vi "ceciLV_tanques.vi"() -> ()   [LabVIEW 2017]
panel:
  out "Tanque B":i64(slide) scale=0.0..100.0
  out "Tanque A":i64(slide) scale=0.0..100.0
  out "Tanque abastecimiento":i64(slide) scale=0.0..200.0
  in  "Presione despues de su seleccion:":bool
  in  "Seleccione el tanque a llenar:":u16(ring) items=["Tanque A", "Tanque B", ""]
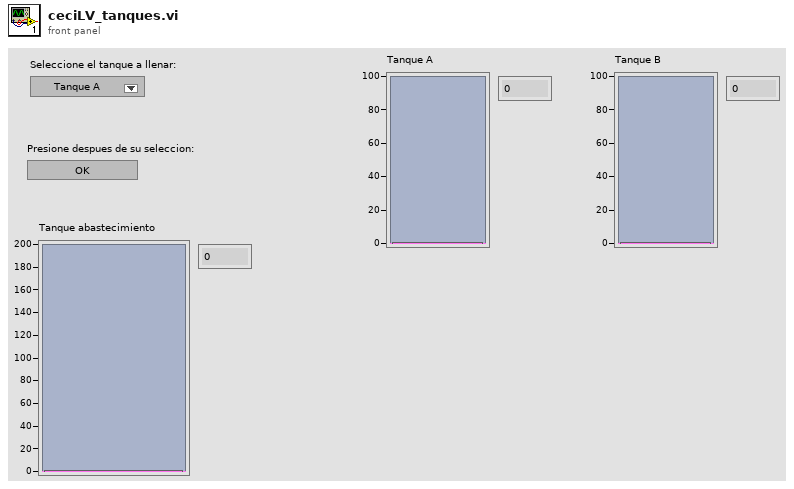
[diagram p1: front panel]
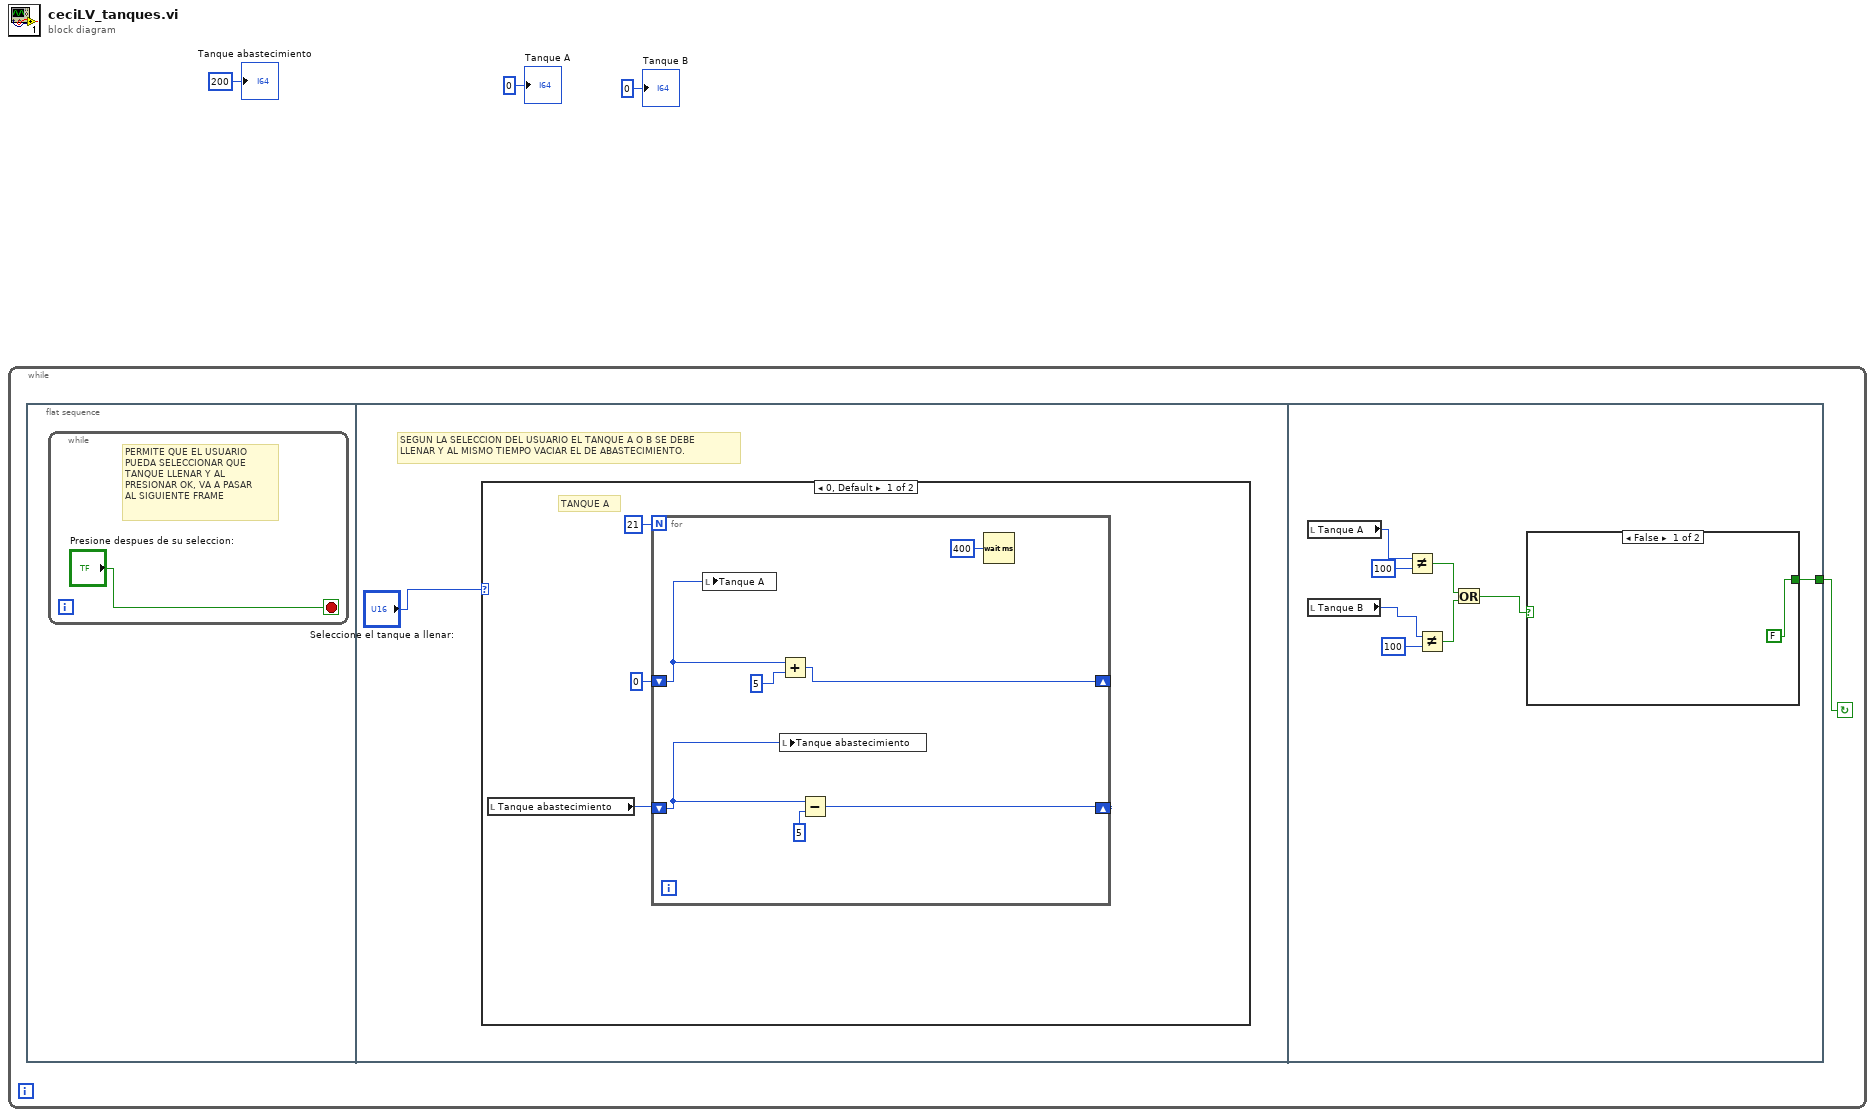
[diagram p0: block diagram]
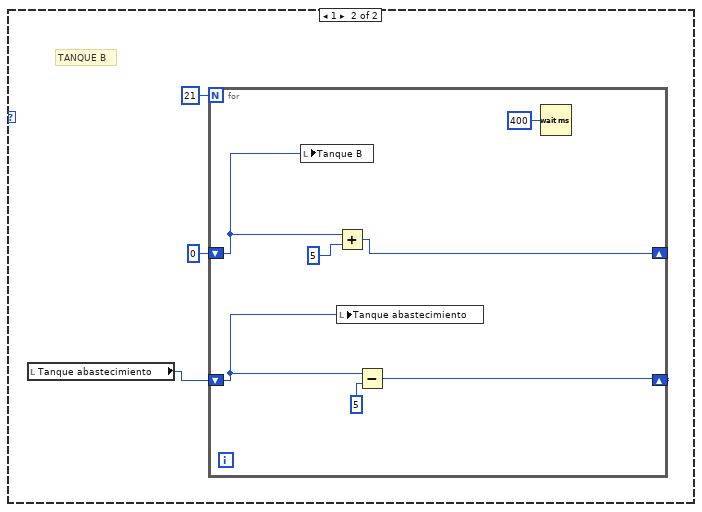
[diagram p2: hidden frame]
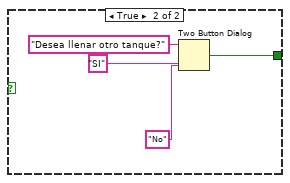
[diagram p3: hidden frame]
diagram:
  n1 = while {
    stop <- w4 continue-if-true
    n2 = flat-sequence {
      tunnel: [w27] -> w4
      frame #0 {
        n3 = while {
          stop <- "Presione despues de su seleccion:" stop-if-true
          # "PERMITE QUE EL USUARIO\nPUEDA SELECCIONAR QUE \nTANQUE LLENAR Y AL \nPRESIONAR OK, VA A PASAR\nAL SIGUIENTE FRAME"
        }
      }
      frame #1 {
        # "SEGUN LA SELECCION DEL USUARIO EL TANQUE A O B SE DEBE \nLLENAR Y AL MISMO TIEMPO VACIAR EL DE ABASTECIMIENTO."
        n4 = case shown="0, Default" "Seleccione el tanque a llenar:" {
          frame 0, Default {
            # "TANQUE A"
            n5 = local read "Tanque abastecimiento"() -> (w7:i64)
            n6 = for {
              N: 21 -> [_]
              shift-right: [w16] -> _
              shift-left: i64 0 -> [w14]
              shift-right: [w12] -> _
              shift-left: w7 -> [w11]
              n7 = local write "Tanque A"(w14) -> ()
              n8 = Add(x=w14, y=i64 5) -> (x+y=w16:i64)
              n9 = local write "Tanque abastecimiento"(w11) -> ()
              n10 = Subtract(x=w11, y=i64 5) -> (x-y=w12:i64)
              n11 = Wait (ms)(milliseconds to wait=u32 400) -> ()  [unwired: 1 out]
            }
          }
          frame 1 {
            # "TANQUE B"
            n12 = local read "Tanque abastecimiento"() -> (w19:i64)
            n13 = for {
              N: 21 -> [_]
              shift-right: [w26] -> _
              shift-left: i64 0 -> [w20]
              shift-right: [w23] -> _
              shift-left: w19 -> [w22]
              n14 = local write "Tanque B"(w20) -> ()
              n15 = Add(x=w20, y=i64 5) -> (x+y=w26:i64)
              n16 = local write "Tanque abastecimiento"(w22) -> ()
              n17 = Subtract(x=w22, y=i64 5) -> (x-y=w23:i64)
              n18 = Wait (ms)(milliseconds to wait=u32 400) -> ()  [unwired: 1 out]
            }
          }
        }
      }
      frame #2 {
        n19 = local read "Tanque A"() -> (w34:i64)
        n20 = local read "Tanque B"() -> (w31:i64)
        n21 = Not Equal?(x=w34, y=i64 100) -> (x != y?=w29:bool)
        n22 = Not Equal?(x=w31, y=i64 100) -> (x != y?=w30:bool)
        n23 = Or(x=w29, y=w30) -> (x .or. y?=w28:bool)
        n24 = case shown="False" w28 {
          tunnel: [FALSE ("T button?") w36] -> w27
          frame False {
          }
          frame True {
            n25 = Two Button Dialog(message="Desea llenar otro tanque?", 1:"No" ("F button name (\"Cancel\")"), 2:"SI" ("T button name (\"OK\")")) -> (T button?=w36:bool)
          }
        }
      }
    }
  }
  "Tanque abastecimiento" <- i64 200 ("Tanque abastecimiento")
  "Tanque A" <- i64 0 ("Tanque A")
  "Tanque B" <- i64 0 ("Tanque B")
